vi "Test-UI.vi"() -> ()   [LabVIEW 2011]
uses:
  Output - Cluster b2g2.ctl
  Input - Cluster b2g2.ctl
panel:
  out "FS-2 (T-2) [l]":sgl(slide) scale=0.0..80.0
  out "FS-1 (T-1)  [l]":sgl(slide) scale=0.0..80.0
  out "pH-Wert":cluster{"pHS-1":dbl}(graph)
  out "pHS-1":dbl
  out "MIN!":bool
  out "MAX!":bool
  out "MIN!":bool
  out "MAX!":bool
  out "T-1&2 Füllstandsüberwachung":bool
  out "MR Füllstandsüberwachung":bool
  out "Heizung":bool
  out "Temp Soll [°C]":sgl min=0 max=100 step=0.1 format="%.1g"
  out "Hysterese [°C]":sgl=0.1 min=0.1 max=10 step=0.1 format="%.1g"
  out "Temperaturregelung":cluster{"Temp Soll":sgl, "TS-4":dbl, i32}(graph)
  out "Temperaturregelung":bool
  out "Temp Ist [°C]":sgl format="%.2g"
  out "V-10 (T-1)":bool
  out "V-14 (T-2)":bool
  out "Zulauf":bool
  out "Dosierung Fertig":bool
  out "Menge Ist [l]":sgl
  out "MIN!":bool
  out "MAX!":bool
  out "P-4 Drehzahl [%]":u8
  out "Menge Soll [l]":sgl format="%.1g"
  out "DFS-1 Volumen [l]":sgl format="%.1f"
  out "Durchfluss Ist  [l/min]":sgl format="%.2f"
  out "Durchfluss Soll [l/min]":sgl format="%.1g"
  out "Dosierung":T1(graph)
  out "Dosierung":bool
  out "Überdruckregelung":cluster{"Druck Soll":sgl, "DS-1":dbl, dbl}(graph)
  out "Druck Soll [bar]":sgl min=0 max=10 step=0.1 format="%.1g"
  out "Füllstand Soll [l]":sgl min=0 max=5 step=0.1 format="%.1g"
  out "Überdruckregelung":bool
  out "Füllstandsregelung":cluster{"Füllstand Soll":sgl, "FS-3":dbl, dbl}(graph)
  out "MR Füllstandsregulierung":bool
  out "P-4":bool
  out "Target Log":bool
  out "FS-3 (MR)":sgl(slide) scale=-1.0..6.0
  out "Druck Ist [bar]":sgl format="%#.2g"
  in  "stop":bool
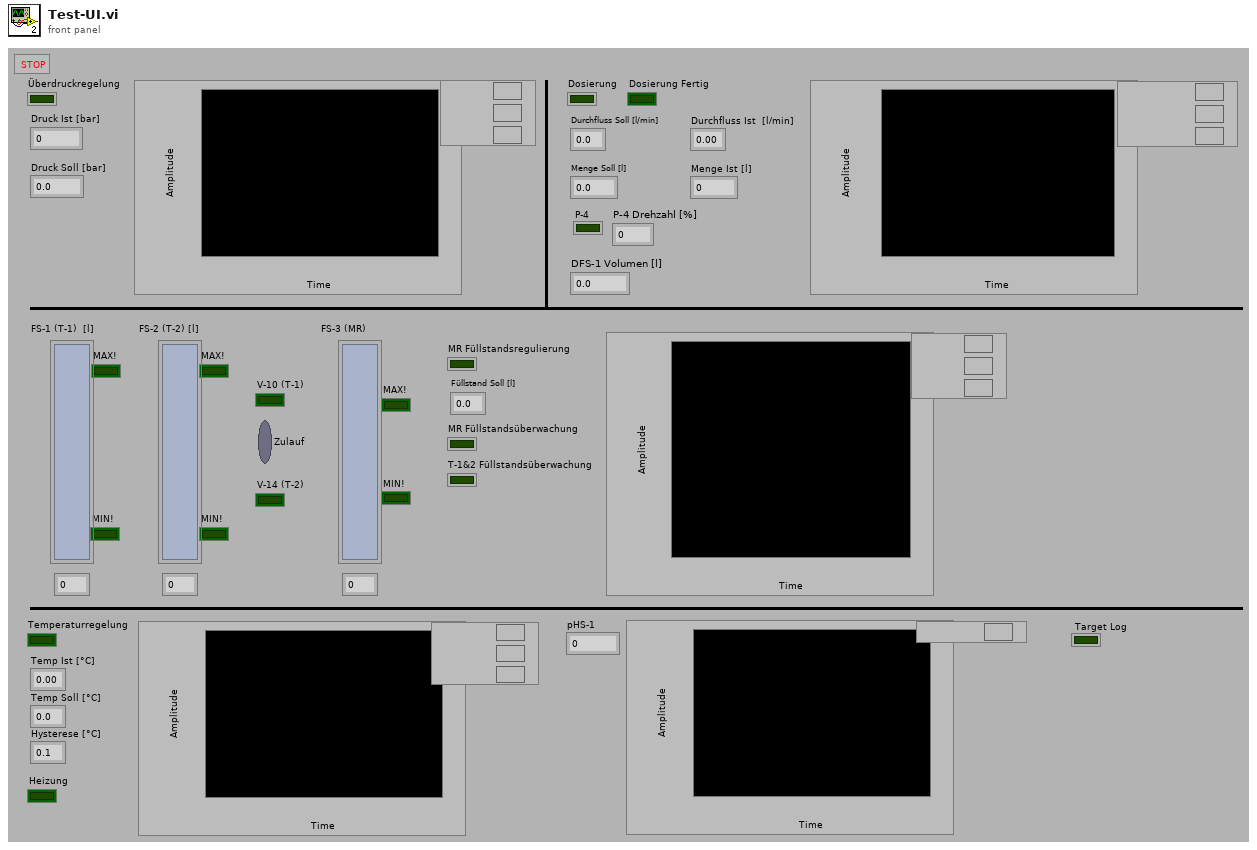
[diagram p1: front panel]
types:
  T1 = cluster{"Dosiergeschwindigkeit [l/min]":sgl, "DFS-1 Durchfluss":dbl, dbl}
  T2 = typedef "Input - Cluster b2g2.ctl" = cluster{"V-13 [%]":u8, "V-15 [%]":u8, "Log-Target":bool, "P-4":bool, "P-4 Drehzahl [%]":u8, "Temperaturregelung":bool, "Überdruckregelung":bool, "Füllstandsregulierung":bool, "V-10":bool, "Log-Host":bool, "V-14":bool, "HS-1":bool, "Füllstand  P":sgl, "Füllstand I":sgl, "Füllstand D":sgl, "Füllstand Soll [l]":sgl, "Druck  P":sgl, "Druck I":sgl, "Druck D":sgl, "Druck Soll [bar]":sgl, "Temp Soll [°C]":sgl, "Dosierung":bool, "Dosiermenge [l]":sgl, "Dosiergeschw. [l/min]":sgl, "Tank":bool, "Hysterese [°C]":sgl, "MR Füllstandsüberwachung":bool, "Tank Füllstandsüberwachung":bool, "Log Target [ms]":u32, "Log Host [s]":u32, "Zirkulation EIN [min]":u8, "Zirkulation AUS [min]":u8, "Zirkulation":bool, "V-33":bool, "V-34":bool, "V-35":bool}
  T3 = typedef "Output - Cluster b2g2.ctl" = cluster{"DFS-1 [dl]":u64, "FS-3 [l]":dbl, "DFS-1 [l/min]":dbl, "DS-1 [bar]":dbl, "V-10 ZU":bool, "V-14 ZU":bool, "FS-1 [l]":dbl, "FS-2 [l]":dbl, "TS-4 [°C]":dbl, "HS-1":bool, "V-13 [%]":u8, "V-15 [%]":u8, "P-4 [%]":u8, "Dosierung":bool, "MR Max Füllstand":bool, "MR Min Füllstand":bool, "Dosiermenge [l]":sgl, "V-14 AUF":bool, "V-10 AUF":bool, "T-1 Max Füllstand":bool, "T-1 Min Füllstand":bool, "T-2 Max Füllstand":bool, "T-2 Min Füllstand":bool, "pHS-1 [pH]":dbl, "P-4 RUN":bool, "V-33 AUF":bool, "V-33 ZU":bool, "V-34 AUF":bool, "V-34 ZU":bool, "P-4 ERR":bool, "TS-5 [°C]":dbl, "V-35 AUF":bool, "V-35 ZU":bool}
  T4 = cluster{"Druck Soll [bar]":sgl, "DS-1 [bar]":dbl, dbl}
  T5 = cluster{"Dosiergeschw. [l/min]":sgl, "DFS-1 [l/min]":dbl, dbl}
  T6 = cluster{"Temp Soll [°C]":sgl, "TS-4 [°C]":dbl, i32}
  T7 = cluster{"Füllstand Soll [l]":sgl, "FS-3 [l]":dbl, dbl}
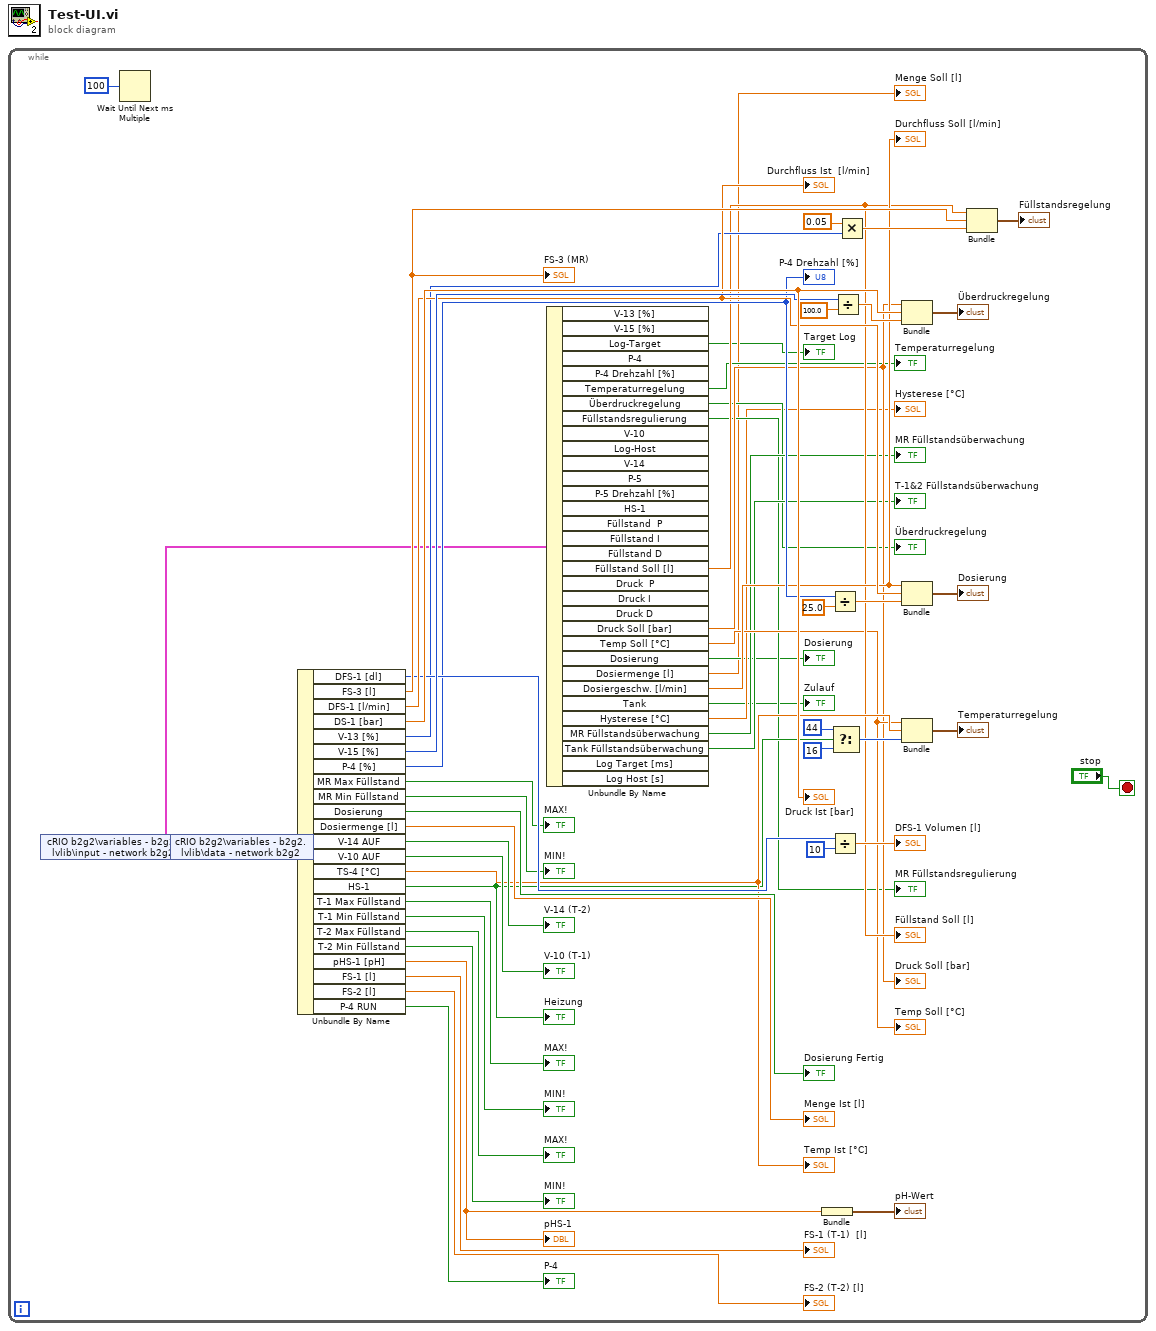
[diagram p0: block diagram]
diagram:
  n1 = while {
    stop <- "stop" stop-if-true
    n2 = shared-variable "cRIO b2g2\\variables - b2g2.lvlib\\input - network b2g2"() -> (w16:T2, error out=w17:errorcluster)  [unwired: 1 in]
    n3 = Wait Until Next ms Multiple(millisecond multiple=u32 100) -> ()  [unwired: 1 out]
    n4 = shared-variable "cRIO b2g2\\variables - b2g2.lvlib\\data - network b2g2"(error in=w17) -> (w30:T3)  [unwired: 1 out]
    n5 = Unbundle By Name(w30) -> ("DFS-1 [dl]"=w49:u64, "FS-3 [l]"=w57:dbl, "DFS-1 [l/min]"=w50:dbl, "DS-1 [bar]"=w55:dbl, "V-13 [%]"=w18:u8, "V-15 [%]"=w53:u8, "P-4 [%]"=w45:u8, "MR Max Füllstand"=→"MAX!":bool, "MR Min Füllstand"=→"MIN!":bool, "Dosierung"=→"Dosierung Fertig":bool, "Dosiermenge [l]"=→"Menge Ist [l]":sgl, "V-14 AUF"=→"V-14 (T-2)":bool, "V-10 AUF"=→"V-10 (T-1)":bool, "TS-4 [°C]"=w37:dbl, "HS-1"=w35:bool, "T-1 Max Füllstand"=→"MAX!":bool, "T-1 Min Füllstand"=→"MIN!":bool, "T-2 Max Füllstand"=→"MAX!":bool, "T-2 Min Füllstand"=→"MIN!":bool, "pHS-1 [pH]"=w24:dbl, "FS-1 [l]"=→"FS-1 (T-1)  [l]":dbl, "FS-2 [l]"=→"FS-2 (T-2) [l]":dbl, "P-4 RUN"=→"P-4":bool)
    "FS-3 (MR)" <- w57
    "Durchfluss Ist  [l/min]" <- w50
    "Druck Ist [bar]" <- w55
    "P-4 Drehzahl [%]" <- w45
    "Temp Ist [°C]" <- w37
    "Heizung" <- w35
    "pHS-1" <- w24
    n6 = Unbundle By Name(w16) -> ("Log-Target"=→"Target Log":bool, "Temperaturregelung"=→"Temperaturregelung":bool, "Überdruckregelung"=→"Überdruckregelung":bool, "Füllstandsregulierung"=→"MR Füllstandsregulierung":bool, "Füllstand Soll [l]"=w14:sgl, "Druck Soll [bar]"=w12:sgl, "Temp Soll [°C]"=w13:sgl, "Dosierung"=→"Dosierung":bool, "Dosiermenge [l]"=→"Menge Soll [l]":sgl, "Dosiergeschw. [l/min]"=w15:sgl, "Tank"=→"Zulauf":bool, "Hysterese [°C]"=→"Hysterese [°C]":sgl, "MR Füllstandsüberwachung"=→"MR Füllstandsüberwachung":bool, "Tank Füllstandsüberwachung"=→"T-1&2 Füllstandsüberwachung":bool)  [unwired: 18 out]
    "Füllstand Soll [l]" <- w14
    "Druck Soll [bar]" <- w12
    "Durchfluss Soll [l/min]" <- w15
    "Temp Soll [°C]" <- w13
    n7 = Bundle("pHS-1 [pH]"=w24) -> (→"pH-Wert":cluster{"pHS-1 [pH]":dbl})  [unwired: 1 in]
    n8 = Divide(x=w45, y=25.0) -> (x/y=w46:dbl)
    n9 = Divide(x=w49, y=u64 10) -> (x/y=→"DFS-1 Volumen [l]":dbl)
    n10 = Select(t=44, s=w35, f=16) -> (s? t:f=w28:i32)
    n11 = Divide(x=w53, y=100.0) -> (x/y=w54:dbl)
    n12 = Multiply(x=0.05, y=w18) -> (x*y=w20:dbl)
    n13 = Bundle("Druck Soll [bar]"=w12, "DS-1 [bar]"=w55, w54) -> (→"Überdruckregelung":T4)  [unwired: 1 in]
    n14 = Bundle("Dosiergeschw. [l/min]"=w15, "DFS-1 [l/min]"=w50, w46) -> (→"Dosierung":T5)  [unwired: 1 in]
    n15 = Bundle("Temp Soll [°C]"=w13, "TS-4 [°C]"=w37, w28) -> (→"Temperaturregelung":T6)  [unwired: 1 in]
    n16 = Bundle("Füllstand Soll [l]"=w14, "FS-3 [l]"=w57, w20) -> (→"Füllstandsregelung":T7)  [unwired: 1 in]
  }
